vi "Configure Filter.vi"(0 "VISA resource name":refnum<visa-resource-name>, 1 "BBT Parameter (0.5)":dbl=0.5, 2 "Alpha Value (0.35)":dbl=0.35, 5 "Modulation Format (0: Custom)":u16(ring) items=["Custom", "Dual Modulation"], 7 "Filter Type (0: Root Nyquist)":u16(ring) items=["Root Nyquist", "Nyquist", "Gaussian", "Rectangle", "IS-95", "IS-95 w/EQ", "IS-95 Mod", "IS-95 Mod w/EQ", "WCDMA", "IS-2000 SR3 DS", "APCO 25 C4FM", "UN3/4 GSM Gaussian", "User FIR"], 9 "File Name (\"\")":string, 11 "error in (no error)":errorcluster, 12 "Optimization Type (0: ACP)":u16(ring) items=["ACP", "EVM"]) -> (4 "VISA resource name out":refnum<visa-resource-name>, 15 "error out":errorcluster)   [LabVIEW 2009, in "Agilent PSG MXG Series.lvlib"]
doc: "Configures the filter for the specific modulation format.\n\n<B>Notes:</B>\n(1) This VI is valid only in E8267C, E8267D, N5182A.\n\n(2) For E8267C, this VI is valid only when the instrument installs <B>Option 002</B> (Internal baseband generator) or <B>Option 602</B> (Digital bus baseband generator).\n\n(3) For E8267D, this VI is valid only when the instrument installs <B>Option 601</B> or <B>Option 602</B> (Internal baseband generator).\n\n(4) For N5182A, this VI is valid only when the instrument installs <B>Option 651</B> or <B>Option 652</B> or <B>Option 654</B> (Internal baseband generator)."
uses:
  Agilent PSG MXG Series.lvlib
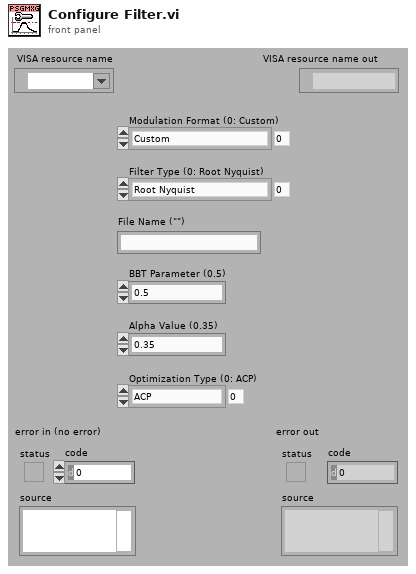
[diagram p1: front panel]
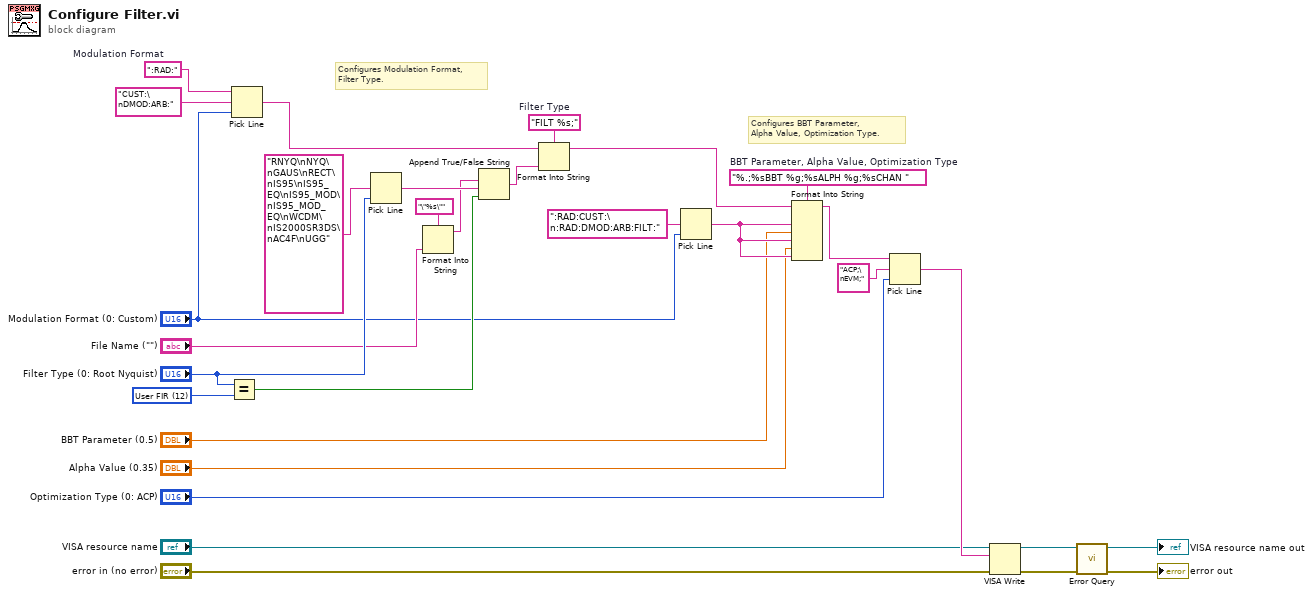
[diagram p0: block diagram]
diagram:
  w15 = "%.;%sBBT %g;%sALPH %g;%sCHAN "  # BBT Parameter, Alpha Value, Optimization Type
  w24 = u16 12 items=["Root Nyquist", "Nyquist", "Gaussian", "Rectangle", "IS-95", "IS-95 w/EQ", "IS-95 Mod", "IS-95 Mod w/EQ", "WCDMA", "IS-2000 SR3 DS", "APCO 25 C4FM", "UN3/4 GSM Gaussian", "User FIR"] ("Filter Type (0: Root Nyquist)")
  w27 = "FILT %s;"  # Filter Type
  w30 = ":RAD:"  # Modulation Format
  # "Configures BBT Parameter,\nAlpha Value, Optimization Type."
  # "Configures Modulation Format,\nFilter Type."
  n1 = Equal?(x="Filter Type (0: Root Nyquist)", y=w24) -> (x = y?=w21:bool)
  n2 = Pick Line(string ("")=w30, multi-line string="CUST:\nDMOD:ARB:", line index="Modulation Format (0: Custom)") -> (output string=w28:string)
  n3 = Pick Line(multi-line string="RNYQ\nNYQ\nGAUS\nRECT\nIS95\nIS95_EQ\nIS95_MOD\nIS95_MOD_EQ\nWCDM\nIS2000SR3DS\nAC4F\nUGG", line index="Filter Type (0: Root Nyquist)") -> (output string=w22:string)  [unwired: 1 out]
  n4 = Format Into String(format string="\"%s\"", "File Name (\"\")") -> (resulting string=w18:string)  [unwired: 2 in, 1 out]
  n5 = Append True/False String(1:w21, 2:w22, 3:w18) -> (0:w23:string)  [unwired: 1 out]
  n6 = Format Into String(format string=w27, initial string=w28, w23) -> (resulting string=w7:string)  [unwired: 1 in, 1 out]
  n7 = Pick Line(multi-line string=":RAD:CUST:\n:RAD:DMOD:ARB:FILT:", line index="Modulation Format (0: Custom)") -> (output string=w8:string)  [unwired: 1 out]
  n8 = Format Into String(format string=w15, initial string=w7, w8, "BBT Parameter (0.5)", w8, "Alpha Value (0.35)", w8) -> (resulting string=w14:string)  [unwired: 1 in, 1 out]
  n9 = Pick Line(string ("")=w14, multi-line string="ACP;\nEVM;", line index="Optimization Type (0: ACP)") -> (output string=w11:string)
  n10 = VISA Write(VISA resource name="VISA resource name", write buffer=w11, error in (no error)="error in (no error)") -> (VISA resource name out=w10:refnum<visa-resource-name>, error out=w9:errorcluster)  [unwired: 1 out]
  n11 = call "Error Query.vi"("error in (no error)"=w9, "VISA resource name"=w10) -> ("error out"=→"error out":errorcluster, "VISA resource name out"=→"VISA resource name out":refnum<visa-resource-name>)  [unwired: 8 out]
